vi "assembly type to channel classification.vi"(11 "Type":T1) -> (3 "channel classification":T2)   [LabVIEW 2013, in "EIP Tags Channel.lvclass"]
uses:
  EIP Tags Channel.lvclass
  <vilib>/NI/Tag Bus Module Framework/channel/channel classification.ctl
  configuration/assembly type.ctl
  <vilib>/NI/Tag Bus Module Framework/channel/TBM channel.lvclass
  configuration/EIP Tags Configuration.lvclass
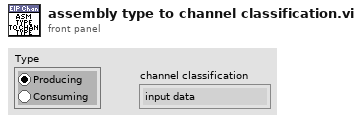
[diagram p1: front panel]
types:
  T1 = typedef "EIP Tags Configuration.lvclass/assembly type.ctl" = enum32{"Producing", "Consuming"}
  T2 = typedef "TBM channel.lvclass/channel classification.ctl" = enum16{"input data", "output data", "processing parameter", "processing result"}
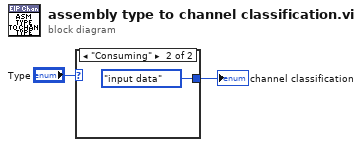
[diagram p0: block diagram]
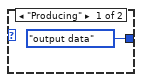
[diagram p2: hidden frame]
diagram:
  n1 = case shown="\"Consuming\"" "Type" {
    tunnel: [channel_classification."output data" ("channel classification") channel_classification."input data" ("channel classification")] -> w2
    frame "Producing" {
    }
    frame "Consuming" {
    }
  }
  "channel classification" <- w2
